vi "TOOLweb SET.vi"(4 "error in (no error)":errorcluster, 5 "IP-Adresse (localhost)":string="127.0.0.1", 6 "Wert-String":string, 7 "EVID-Nummer":i32=1) -> (0 "error out":errorcluster, 2 "Neuer Wert":string, 3 "Feedback":i32)   [LabVIEW 2020, in "FT-IR.lvlib" / "TOOLweb Interface.lvlib"]
doc: "Setzt den Wert der Variablen \"EVID-Nummer\" auf den neuen Wert \"Wert-String\". \nDer Integer-Ausgang \"Feedback\" gibt Auskunft über die erfolgreiche Ausführung des Set-Requests, wobei nur der Wert 0 (=success) für alle EVIDs gleich ist. Fehlermeldungen in Form einer Feedback-Zahl ungleich Null variieren und müssen mit dem Handbuch des Gas-Analysators interpretiert werden.\nDer String \"Neuer Wert\" enthält den EVID-Wert nach Ausführung des Set-Requests. \n\nFalls der TOOLWeb-Server nicht auf demselben Rechner arbeitet, kann mit \"IP-Adresse\" eine beliebiger Host adressiert werden. Ein unverbundener Eingang spricht den lokalen Host an."
uses:
  TOOLweb Interface.lvlib
  TOOLweb Interface Hilfs-VIs.lvlib
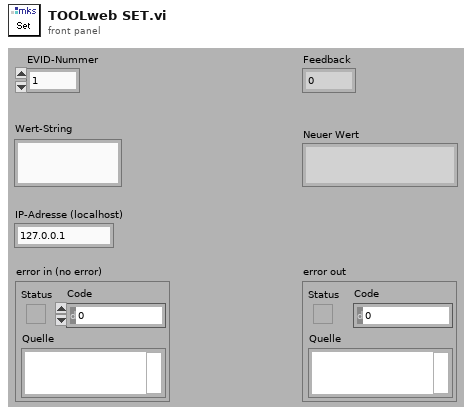
[diagram p1: front panel]
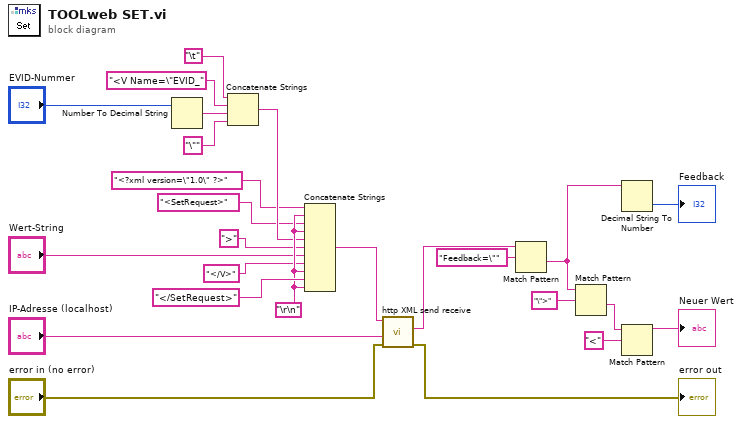
[diagram p0: block diagram]
diagram:
  w13 = "\r\n"
  n1 = Number To Decimal String(number="EVID-Nummer") -> (decimal integer string=w5:string)  [unwired: 1 out]
  n2 = Concatenate Strings("\t", "<V Name=\"EVID_" ("Daten (Eingang)"), w5, "\"" ("Daten (Eingang)")) -> (w9:string)
  n3 = Concatenate Strings("<?xml version=\"1.0\" ?>" ("Daten (Eingang)"), w13, "<SetRequest>" ("Daten (Eingang)"), w13, w9, ">" ("Daten (Eingang)"), "Wert-String", "</V>" ("Daten (Eingang)"), w13, "</SetRequest>" ("Daten (Eingang)"), w13) -> (w2:string)
  n4 = call "http XML send receive.vi"("error in (no error)"="error in (no error)", "IP-Adresse (localhost)"="IP-Adresse (localhost)", "XML Request"=w2) -> ("error out"=→"error out":errorcluster, "Response Body (XML)"=w1:string)  [unwired: 3 out]
  n5 = Match Pattern(string=w1, regular expression="Feedback=\"" ("Regulärer Ausdruck")) -> (after substring=w20:string)  [unwired: 4 out]
  n6 = Match Pattern(string=w20, regular expression="\">" ("Regulärer Ausdruck")) -> (after substring=w17:string)  [unwired: 4 out]
  n7 = Decimal String To Number(string=w20) -> (number=→"Feedback":i32)  [unwired: 3 out]
  n8 = Match Pattern(string=w17, regular expression="<" ("Regulärer Ausdruck")) -> (before substring=→"Neuer Wert":string)  [unwired: 4 out]
